vi "Numeric Travel to Formatted String.vi"(6 "Travel Units":T1, 8 "error in (no error)":errorcluster, 9 "Travel Direction":T2, 10 "Travel":dbl format="%.3f", 11 "ESM303 in":refnum<class "ESM303.lvclass">) -> (0 "error out":errorcluster, 2 "Formatted Travel String":string, 3 "ESM303 out":refnum<class "ESM303.lvclass">)   [LabVIEW 2018, in "ESM303.lvlib" / "ESM303.lvclass"]
uses:
  ESM303.lvclass
  builds/Force Test Stand/Force Test Stand/Force Test Stand.lvlibp/Custom Controls/Travel Direction.ctl
  builds/Force Test Stand/Force Test Stand/Force Test Stand.lvlibp/Custom Controls/Travel Units.ctl
  builds/Force Test Stand/Force Test Stand/Force Test Stand.lvlibp/Force Test Stand.lvclass
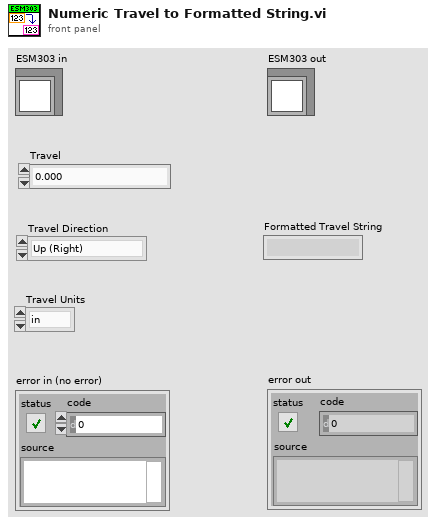
[diagram p1: front panel]
types:
  T1 = typedef "Force Test Stand.lvlibp/Force Test Stand.lvclass/Travel Units.ctl" = enum16{"in", "mm"}
  T2 = typedef "Force Test Stand.lvlibp/Force Test Stand.lvclass/Travel Direction.ctl" = enum16{"Up (Right)", "Down (Left)"}
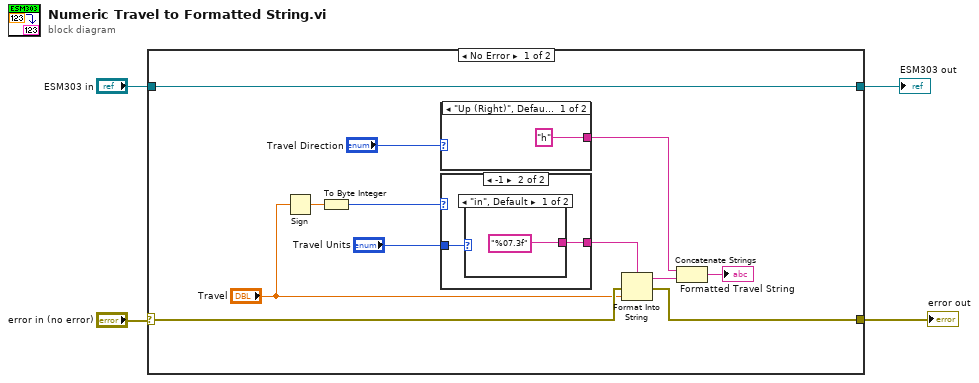
[diagram p0: block diagram]
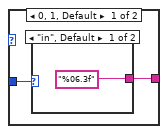
[diagram p2: hidden frame]
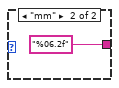
[diagram p3: hidden frame]
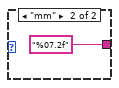
[diagram p4: hidden frame]
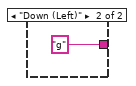
[diagram p5: hidden frame]
diagram:
  n1 = case shown="No Error" "error in (no error)" {
    selector: "error in (no error)" -> [w13 w27]
    tunnel: [w15 w28] -> w4
    tunnel: "ESM303 in" -> [w15 w28]
    tunnel: [w12 w27] -> w1
    frame No Error {
      n2 = Sign(1:"Travel") -> (0:w8:dbl)
      n3 = To Byte Integer(number=w8) -> (8bit integer=w7:i8)
      n4 = case shown="\"Up (Right)\", Default" "Travel Direction" {
        tunnel: ["h" "g"] -> w10
        frame "Up (Right)", Default {
        }
        frame "Down (Left)" {
        }
      }
      n5 = case shown="-1" w7 {
        tunnel: "Travel Units" -> [w18 w21]
        tunnel: [w17 w22] -> w5
        frame 0, 1, Default {
          n6 = case shown="\"in\", Default" w18 {
            tunnel: ["%06.3f" ("format string") "%06.2f" ("format string")] -> w17
            frame "in", Default {
            }
            frame "mm" {
            }
          }
        }
        frame -1 {
          n7 = case shown="\"in\", Default" w21 {
            tunnel: ["%07.3f" ("format string") "%07.2f" ("format string")] -> w22
            frame "in", Default {
            }
            frame "mm" {
            }
          }
        }
      }
      n8 = Format Into String(format string=w5, error in=w13, "Travel") -> (resulting string=w16:string, error out=w12:errorcluster)  [unwired: 1 in]
      n9 = Concatenate Strings(w10, w16) -> (→"Formatted Travel String":string)
    }
    frame Error {
    }
  }
  "error out" <- w1
  "ESM303 out" <- w4
